vi "Find Header Value.vi"   [LabVIEW 2020, in "Blue Easy HTTP OpenSource.lvlib"]
uses:
  Blue Easy HTTP OpenSource.lvlib
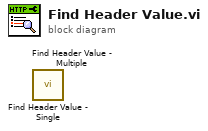
[diagram p0: block diagram]
diagram:
  n1 = call "Find Header Value - Single.vi"() -> ()  [unwired: 9 in, 3 out]
  n2 = call "Find Header Value - Multiple.vi"() -> ()  [unwired: 9 in, 3 out]
